vi "kickout_some_PVs_fromLINAC.vi"() -> ()   [LabVIEW 2013]
panel:
  out "Array 2":i32[][](array[numeric])
  out "size(s) 3":i32
  out "size(s) 2":i32
  out "size(s)":i32
  out "Array":string[](array[string])
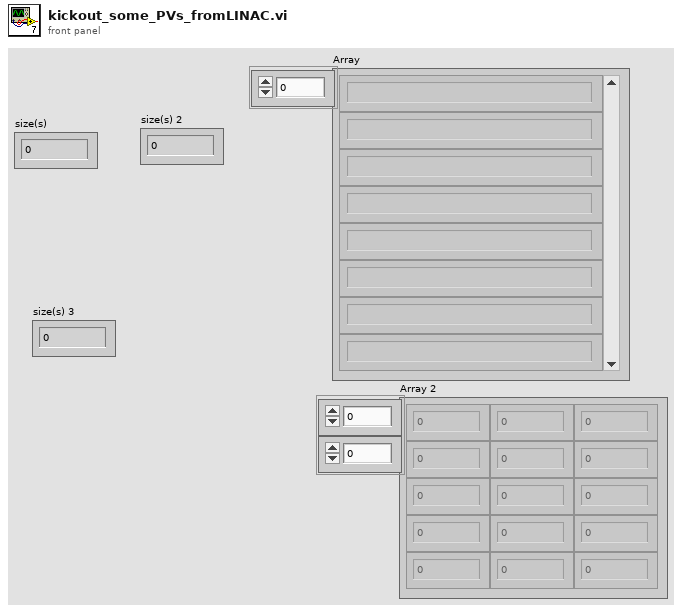
[diagram p1: front panel]
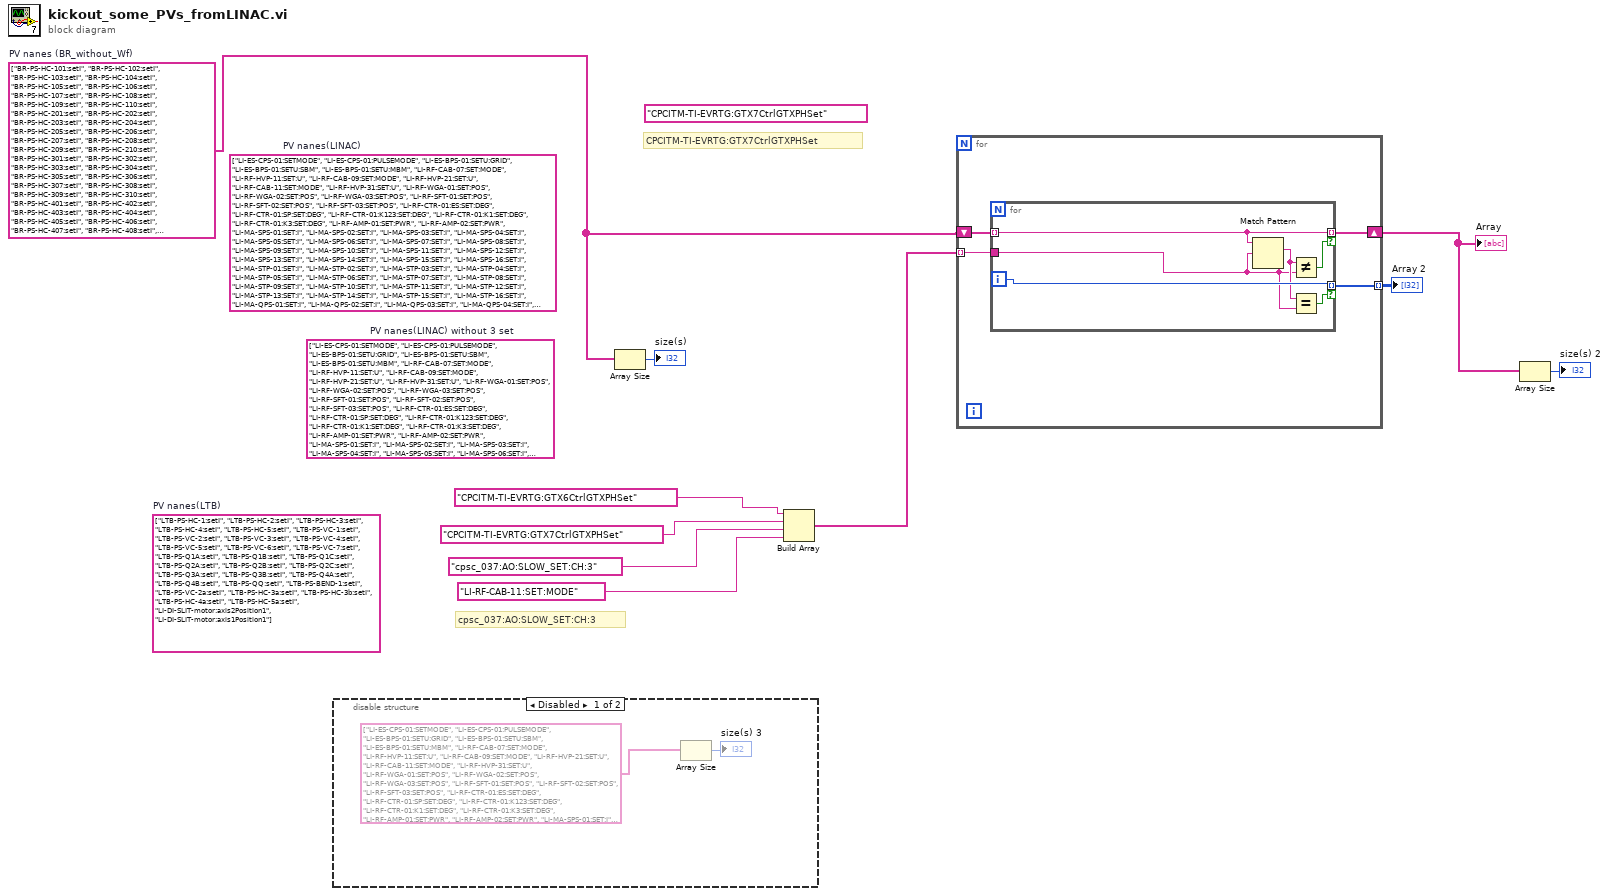
[diagram p0: block diagram]
diagram:
  w1 = string[] ["BR-PS-HC-101:setI", "BR-PS-HC-102:setI", "BR-PS-HC-103:setI", "BR-PS-HC-104:setI", "BR-PS-HC-105:setI", "BR-PS-HC-106:setI", "BR-PS-HC-107:setI", "BR-PS-HC-108:setI", "BR-PS-HC-109:setI", "BR-PS-HC-110:setI", "BR-PS-HC-201:setI", "BR-PS-HC-202:setI", "BR-PS-HC-203:setI", "BR-PS-HC-204:setI", "BR-PS-HC-205:setI", "BR-PS-HC-206:setI", "BR-PS-HC-207:setI", "BR-PS-HC-208:setI", "BR-PS-HC-209:setI", "BR-PS-HC-210:setI", "BR-PS-HC-301:setI", "BR-PS-HC-302:setI", "BR-PS-HC-303:setI", "BR-PS-HC-304:setI", "BR-PS-HC-305:setI", "BR-PS-HC-306:setI", "BR-PS-HC-307:setI", "BR-PS-HC-308:setI", "BR-PS-HC-309:setI", "BR-PS-HC-310:setI", "BR-PS-HC-401:setI", "BR-PS-HC-402:setI", "BR-PS-HC-403:setI", "BR-PS-HC-404:setI", "BR-PS-HC-405:setI", "BR-PS-HC-406:setI", "BR-PS-HC-407:setI", "BR-PS-HC-408:setI", "BR-PS-HC-409:setI", "BR-PS-HC-410:setI", "BR-PS-HC-501:setI", "BR-PS-HC-502:setI", "BR-PS-HC-503:setI", "BR-PS-HC-504:setI", "BR-PS-HC-505:setI", "BR-PS-HC-506:setI", "BR-PS-HC-507:setI", "BR-PS-HC-508:setI", "BR-PS-HC-509:setI", "BR-PS-HC-510:setI", "BR-PS-HC-601:setI", "BR-PS-HC-602:setI", "BR-PS-HC-603:setI", "BR-PS-HC-603a:setI", "BR-PS-HC-604:setI", "BR-PS-HC-605:setI", "BR-PS-HC-606:setI", "BR-PS-HC-606a:setI", "BR-PS-HC-607:setI", "BR-PS-HC-608:setI", "BR-PS-HC-609:setI", "BR-PS-HC-610:setI", "BR-PS-VC-101:setI", "BR-PS-VC-102:setI", "BR-PS-VC-103:setI", "BR-PS-VC-104:setI", "BR-PS-VC-105:setI", "BR-PS-VC-106:setI", "BR-PS-VC-201:setI", "BR-PS-VC-202:setI", "BR-PS-VC-203:setI", "BR-PS-VC-204:setI", "BR-PS-VC-205:setI", "BR-PS-VC-206:setI", "BR-PS-VC-301:setI", "BR-PS-VC-302:setI", "BR-PS-VC-303:setI", "BR-PS-VC-304:setI", "BR-PS-VC-305:setI", "BR-PS-VC-306:setI", "BR-PS-VC-401:setI", "BR-PS-VC-402:setI", "BR-PS-VC-403:setI", "BR-PS-VC-404:setI", "BR-PS-VC-405:setI", "BR-PS-VC-406:setI", "BR-PS-VC-501:setI", "BR-PS-VC-502:setI", "BR-PS-VC-503:setI", "BR-PS-VC-504:setI", "BR-PS-VC-505:setI", "BR-PS-VC-506:setI", "BR-PS-VC-601:setI", "BR-PS-VC-602:setI", "BR-PS-VC-602a:setI", "BR-PS-VC-603:setI", "BR-PS-VC-604:setI", "BR-PS-VC-604a:setI", "BR-PS-VC-605:setI", "BR-PS-VC-606:setI", "BR-PS-VC-100a:setI", "BR-PS-SD:setI", "BR-PS-SF:setI", "cpsc_027:AO:SLOW_SET:CH:1", "cpsc_037:AO:SLOW_SET:CH:3", "BR-RF-LLRF:setStationPhase", "TI-INJ-PROC:setTinj", "BR-PS-INJ-SE:setHV", "CPCIPM-TI-EVR:Pulse1DelaySet", "BR-PS-INJ-KI:setHV", "CPCIPM-TI-EVR:Pulse2DelaySet", "BR-PS-QF:setWfDC", "BR-PS-QM:setWfDC", "BR-PS-Q1:setWfDC", "BR-PS-Q2:setWfDC", "BR-PS-BEND:setWfDC"]  # PV nanes (BR_without_Wf)
  (unwired) string[] ["LTB-PS-HC-1:setI", "LTB-PS-HC-2:setI", "LTB-PS-HC-3:setI", "LTB-PS-HC-4:setI", "LTB-PS-HC-5:setI", "LTB-PS-VC-1:setI", "LTB-PS-VC-2:setI", "LTB-PS-VC-3:setI", "LTB-PS-VC-4:setI", "LTB-PS-VC-5:setI", "LTB-PS-VC-6:setI", "LTB-PS-VC-7:setI", "LTB-PS-Q1A:setI", "LTB-PS-Q1B:setI", "LTB-PS-Q1C:setI", "LTB-PS-Q2A:setI", "LTB-PS-Q2B:setI", "LTB-PS-Q2C:setI", "LTB-PS-Q3A:setI", "LTB-PS-Q3B:setI", "LTB-PS-Q4A:setI", "LTB-PS-Q4B:setI", "LTB-PS-QQ:setI", "LTB-PS-BEND-1:setI", "LTB-PS-VC-2a:setI", "LTB-PS-HC-3a:setI", "LTB-PS-HC-3b:setI", "LTB-PS-HC-4a:setI", "LTB-PS-HC-5a:setI", "LI-DI-SLIT-motor:axis2Position1", "LI-DI-SLIT-motor:axis1Position1"]  # PV nanes(LTB)
  (unwired) string[] ["LI-ES-CPS-01:SETMODE", "LI-ES-CPS-01:PULSEMODE", "LI-ES-BPS-01:SETU:GRID", "LI-ES-BPS-01:SETU:SBM", "LI-ES-BPS-01:SETU:MBM", "LI-RF-CAB-07:SET:MODE", "LI-RF-HVP-11:SET:U", "LI-RF-CAB-09:SET:MODE", "LI-RF-HVP-21:SET:U", "LI-RF-HVP-31:SET:U", "LI-RF-WGA-01:SET:POS", "LI-RF-WGA-02:SET:POS", "LI-RF-WGA-03:SET:POS", "LI-RF-SFT-01:SET:POS", "LI-RF-SFT-02:SET:POS", "LI-RF-SFT-03:SET:POS", "LI-RF-CTR-01:ES:SET:DEG", "LI-RF-CTR-01:SP:SET:DEG", "LI-RF-CTR-01:K123:SET:DEG", "LI-RF-CTR-01:K1:SET:DEG", "LI-RF-CTR-01:K3:SET:DEG", "LI-RF-AMP-01:SET:PWR", "LI-RF-AMP-02:SET:PWR", "LI-MA-SPS-01:SET:I", "LI-MA-SPS-02:SET:I", "LI-MA-SPS-03:SET:I", "LI-MA-SPS-04:SET:I", "LI-MA-SPS-05:SET:I", "LI-MA-SPS-06:SET:I", "LI-MA-SPS-07:SET:I", "LI-MA-SPS-08:SET:I", "LI-MA-SPS-09:SET:I", "LI-MA-SPS-10:SET:I", "LI-MA-SPS-11:SET:I", "LI-MA-SPS-12:SET:I", "LI-MA-SPS-13:SET:I", "LI-MA-SPS-14:SET:I", "LI-MA-SPS-15:SET:I", "LI-MA-SPS-16:SET:I", "LI-MA-STP-01:SET:I", "LI-MA-STP-02:SET:I", "LI-MA-STP-03:SET:I", "LI-MA-STP-04:SET:I", "LI-MA-STP-05:SET:I", "LI-MA-STP-06:SET:I", "LI-MA-STP-07:SET:I", "LI-MA-STP-08:SET:I", "LI-MA-STP-09:SET:I", "LI-MA-STP-10:SET:I", "LI-MA-STP-11:SET:I", "LI-MA-STP-12:SET:I", "LI-MA-STP-13:SET:I", "LI-MA-STP-14:SET:I", "LI-MA-STP-15:SET:I", "LI-MA-STP-16:SET:I", "LI-MA-QPS-01:SET:I", "LI-MA-QPS-02:SET:I", "LI-MA-QPS-03:SET:I", "LI-MA-QPS-04:SET:I", "LI-MA-QPS-05:SET:I", "LI-MA-QPS-06:SET:I", "CPCITM-TI-EVRTG:Pulse7DelaySet", "CPCITM-TI-EVRTG:Pulse7WidthSet", "CPCITM-TI-EVRTG:GTX7DlySet", "CPCITM-TI-EVRTG:Pulse6DelaySet", "CPCITM-TI-EVRTG:Pulse6WidthSet", "CPCITM-TI-EVRTG:GTX6DlySet", "CPCILI-TI-EVR:Pulse2DelaySet", "CPCILI-TI-EVR:Pulse2WidthSet", "CPCILI-TI-EVR:Pulse3DelaySet", "CPCILI-TI-EVR:Pulse3WidthSet", "CPCILI-TI-EVR:Pulse4DelaySet", "CPCILI-TI-EVR:Pulse4WidthSet", "CPCILI-TI-EVR:Pulse5DelaySet", "CPCILI-TI-EVR:Pulse5WidthSet", "CPCILI-TI-EVR:Pulse6DelaySet", "CPCILI-TI-EVR:Pulse6WidthSet", "CPCILI-TI-EVR:Pulse7DelaySet", "CPCILI-TI-EVR:Pulse7WidthSet", "CPCILI-TI-EVR:Pulse8DelaySet", "CPCILI-TI-EVR:Pulse8WidthSet", "CPCILI-TI-EVR:Pulse9DelaySet", "CPCILI-TI-EVR:Pulse9WidthSet", "CPCITM-TI-EVRTG:GTX6DlySet", "CPCITM-TI-EVRTG:GTX7DlySet"]  # PV nanes(LINAC) without 3 set
  (unwired) "CPCITM-TI-EVRTG:GTX7CtrlGTXPHSet" ("regular expression")
  (unwired) string[] ["LI-ES-CPS-01:SETMODE", "LI-ES-CPS-01:PULSEMODE", "LI-ES-BPS-01:SETU:GRID", "LI-ES-BPS-01:SETU:SBM", "LI-ES-BPS-01:SETU:MBM", "LI-RF-CAB-07:SET:MODE", "LI-RF-HVP-11:SET:U", "LI-RF-CAB-09:SET:MODE", "LI-RF-HVP-21:SET:U", "LI-RF-CAB-11:SET:MODE", "LI-RF-HVP-31:SET:U", "LI-RF-WGA-01:SET:POS", "LI-RF-WGA-02:SET:POS", "LI-RF-WGA-03:SET:POS", "LI-RF-SFT-01:SET:POS", "LI-RF-SFT-02:SET:POS", "LI-RF-SFT-03:SET:POS", "LI-RF-CTR-01:ES:SET:DEG", "LI-RF-CTR-01:SP:SET:DEG", "LI-RF-CTR-01:K123:SET:DEG", "LI-RF-CTR-01:K1:SET:DEG", "LI-RF-CTR-01:K3:SET:DEG", "LI-RF-AMP-01:SET:PWR", "LI-RF-AMP-02:SET:PWR", "LI-MA-SPS-01:SET:I", "LI-MA-SPS-02:SET:I", "LI-MA-SPS-03:SET:I", "LI-MA-SPS-04:SET:I", "LI-MA-SPS-05:SET:I", "LI-MA-SPS-06:SET:I", "LI-MA-SPS-07:SET:I", "LI-MA-SPS-08:SET:I", "LI-MA-SPS-09:SET:I", "LI-MA-SPS-10:SET:I", "LI-MA-SPS-11:SET:I", "LI-MA-SPS-12:SET:I", "LI-MA-SPS-13:SET:I", "LI-MA-SPS-14:SET:I", "LI-MA-SPS-15:SET:I", "LI-MA-SPS-16:SET:I", "LI-MA-STP-01:SET:I", "LI-MA-STP-02:SET:I", "LI-MA-STP-03:SET:I", "LI-MA-STP-04:SET:I", "LI-MA-STP-05:SET:I", "LI-MA-STP-06:SET:I", "LI-MA-STP-07:SET:I", "LI-MA-STP-08:SET:I", "LI-MA-STP-09:SET:I", "LI-MA-STP-10:SET:I", "LI-MA-STP-11:SET:I", "LI-MA-STP-12:SET:I", "LI-MA-STP-13:SET:I", "LI-MA-STP-14:SET:I", "LI-MA-STP-15:SET:I", "LI-MA-STP-16:SET:I", "LI-MA-QPS-01:SET:I", "LI-MA-QPS-02:SET:I", "LI-MA-QPS-03:SET:I", "LI-MA-QPS-04:SET:I", "LI-MA-QPS-05:SET:I", "LI-MA-QPS-06:SET:I", "CPCITM-TI-EVRTG:Pulse7DelaySet", "CPCITM-TI-EVRTG:Pulse7WidthSet", "CPCITM-TI-EVRTG:GTX7CtrlGTXPHSet", "CPCITM-TI-EVRTG:GTX7DlySet", "CPCITM-TI-EVRTG:Pulse6DelaySet", "CPCITM-TI-EVRTG:Pulse6WidthSet", "CPCITM-TI-EVRTG:GTX6CtrlGTXPHSet", "CPCITM-TI-EVRTG:GTX6DlySet", "CPCILI-TI-EVR:Pulse2DelaySet", "CPCILI-TI-EVR:Pulse2WidthSet", "CPCILI-TI-EVR:Pulse3DelaySet", "CPCILI-TI-EVR:Pulse3WidthSet", "CPCILI-TI-EVR:Pulse4DelaySet", "CPCILI-TI-EVR:Pulse4WidthSet", "CPCILI-TI-EVR:Pulse5DelaySet", "CPCILI-TI-EVR:Pulse5WidthSet", "CPCILI-TI-EVR:Pulse6DelaySet", "CPCILI-TI-EVR:Pulse6WidthSet", "CPCILI-TI-EVR:Pulse7DelaySet", "CPCILI-TI-EVR:Pulse7WidthSet", "CPCILI-TI-EVR:Pulse8DelaySet", "CPCILI-TI-EVR:Pulse8WidthSet", "CPCILI-TI-EVR:Pulse9DelaySet", "CPCILI-TI-EVR:Pulse9WidthSet", "CPCITM-TI-EVRTG:GTX6DlySet", "CPCITM-TI-EVRTG:GTX7DlySet"]  # PV nanes(LINAC)
  # "cpsc_037:AO:SLOW_SET:CH:3"
  # "CPCITM-TI-EVRTG:GTX7CtrlGTXPHSet"
  n1 = disable-structure shown="Disabled" {
    frame Disabled {
      n2 = Array Size(array=string[] ["LI-ES-CPS-01:SETMODE", "LI-ES-CPS-01:PULSEMODE", "LI-ES-BPS-01:SETU:GRID", "LI-ES-BPS-01:SETU:SBM", "LI-ES-BPS-01:SETU:MBM", "LI-RF-CAB-07:SET:MODE", "LI-RF-HVP-11:SET:U", "LI-RF-CAB-09:SET:MODE", "LI-RF-HVP-21:SET:U", "LI-RF-CAB-11:SET:MODE", "LI-RF-HVP-31:SET:U", "LI-RF-WGA-01:SET:POS", "LI-RF-WGA-02:SET:POS", "LI-RF-WGA-03:SET:POS", "LI-RF-SFT-01:SET:POS", "LI-RF-SFT-02:SET:POS", "LI-RF-SFT-03:SET:POS", "LI-RF-CTR-01:ES:SET:DEG", "LI-RF-CTR-01:SP:SET:DEG", "LI-RF-CTR-01:K123:SET:DEG", "LI-RF-CTR-01:K1:SET:DEG", "LI-RF-CTR-01:K3:SET:DEG", "LI-RF-AMP-01:SET:PWR", "LI-RF-AMP-02:SET:PWR", "LI-MA-SPS-01:SET:I", "LI-MA-SPS-02:SET:I", "LI-MA-SPS-03:SET:I", "LI-MA-SPS-04:SET:I", "LI-MA-SPS-05:SET:I", "LI-MA-SPS-06:SET:I", "LI-MA-SPS-07:SET:I", "LI-MA-SPS-08:SET:I", "LI-MA-SPS-09:SET:I", "LI-MA-SPS-10:SET:I", "LI-MA-SPS-11:SET:I", "LI-MA-SPS-12:SET:I", "LI-MA-SPS-13:SET:I", "LI-MA-SPS-14:SET:I", "LI-MA-SPS-15:SET:I", "LI-MA-SPS-16:SET:I", "LI-MA-STP-01:SET:I", "LI-MA-STP-02:SET:I", "LI-MA-STP-03:SET:I", "LI-MA-STP-04:SET:I", "LI-MA-STP-05:SET:I", "LI-MA-STP-06:SET:I", "LI-MA-STP-07:SET:I", "LI-MA-STP-08:SET:I", "LI-MA-STP-09:SET:I", "LI-MA-STP-10:SET:I", "LI-MA-STP-11:SET:I", "LI-MA-STP-12:SET:I", "LI-MA-STP-13:SET:I", "LI-MA-STP-14:SET:I", "LI-MA-STP-15:SET:I", "LI-MA-STP-16:SET:I", "LI-MA-QPS-01:SET:I", "LI-MA-QPS-02:SET:I", "LI-MA-QPS-03:SET:I", "LI-MA-QPS-04:SET:I", "LI-MA-QPS-05:SET:I", "LI-MA-QPS-06:SET:I", "CPCITM-TI-EVRTG:Pulse7DelaySet", "CPCITM-TI-EVRTG:Pulse7WidthSet", "CPCITM-TI-EVRTG:GTX7DlySet", "CPCITM-TI-EVRTG:Pulse6DelaySet", "CPCITM-TI-EVRTG:Pulse6WidthSet", "CPCITM-TI-EVRTG:GTX6DlySet", "CPCILI-TI-EVR:Pulse2DelaySet", "CPCILI-TI-EVR:Pulse2WidthSet", "CPCILI-TI-EVR:Pulse3DelaySet", "CPCILI-TI-EVR:Pulse3WidthSet", "CPCILI-TI-EVR:Pulse4DelaySet", "CPCILI-TI-EVR:Pulse4WidthSet", "CPCILI-TI-EVR:Pulse5DelaySet", "CPCILI-TI-EVR:Pulse5WidthSet", "CPCILI-TI-EVR:Pulse6DelaySet", "CPCILI-TI-EVR:Pulse6WidthSet", "CPCILI-TI-EVR:Pulse7DelaySet", "CPCILI-TI-EVR:Pulse7WidthSet", "CPCILI-TI-EVR:Pulse8DelaySet", "CPCILI-TI-EVR:Pulse8WidthSet", "CPCILI-TI-EVR:Pulse9DelaySet", "CPCILI-TI-EVR:Pulse9WidthSet", "CPCITM-TI-EVRTG:GTX6DlySet", "CPCITM-TI-EVRTG:GTX7DlySet"] ("Array")) -> (size(s)=→"size(s) 3":i32)
    }
    frame Enabled {
    }
  }
  n3 = Array Size(array=w1) -> (size(s)=→"size(s)":i32)
  n4 = Build Array("CPCITM-TI-EVRTG:GTX6CtrlGTXPHSet" ("regular expression"), "CPCITM-TI-EVRTG:GTX7CtrlGTXPHSet" ("regular expression"), "cpsc_037:AO:SLOW_SET:CH:3" ("regular expression"), "LI-RF-CAB-11:SET:MODE" ("element")) -> (w4:string[])
  n5 = for {
    tunnel: w4 -> [w15] mode=indexing
    shift-right: [w16] -> w8
    shift-left: w1 -> [w14]
    tunnel: [w13] -> w2 mode=indexing
    n6 = for {
      tunnel: w14 -> [w22] mode=indexing
      tunnel: [w22] -> w16 mode=indexing if=w21
      tunnel: w15 -> [w18]
      tunnel: [w20] -> w13 mode=indexing if=w17
      i -> [w20]
      n7 = Match Pattern(string=w22, regular expression=w18) -> (match substring=w19:string)  [unwired: 1 in, 3 out]
      n8 = Not Equal?(x=w19, y=w18) -> (x != y?=w21:bool)
      n9 = Equal?(x=w19, y=w18) -> (x = y?=w17:bool)
    }
  }
  "Array" <- w8
  "Array 2" <- w2
  n10 = Array Size(array=w8) -> (size(s)=→"size(s) 2":i32)
